vi "ensureLineFeedAfterString.vi"(8 "error in (no error)":errorcluster, 10 "Element":string, 11 "WriteElement in":refnum<class "XMLGenerator.lvclass">) -> (0 "error out":errorcluster, 2 "ElementWithNewLine":string, 3 "WriteElement out":refnum<class "XMLGenerator.lvclass">)   [LabVIEW 2016, in "XML.lvlib" / "XMLGenerator.lvclass"]
doc: "This method seraches the Element in and returns the element back with a line feed."
uses:
  <userlib>/Common/XML/XMLGenerator/XMLGenerator.lvclass
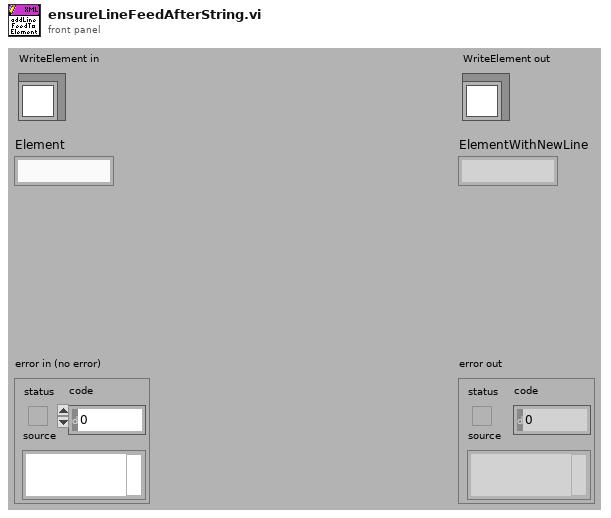
[diagram p1: front panel]
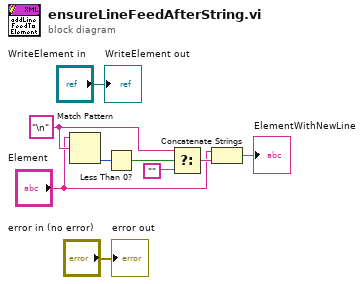
[diagram p0: block diagram]
diagram:
  w3 = "\n" ("regular expression")
  n1 = Match Pattern(string="Element", regular expression=w3) -> (offset past match=w7:i32)  [unwired: 1 in, 3 out]
  n2 = Less Than 0?(x=w7) -> (x < 0?=w6:bool)
  n3 = Select(t=w3, s=w6, f="") -> (s? t:f=w5:string)
  n4 = Concatenate Strings("Element", w5) -> (→"ElementWithNewLine":string)
  "error out" <- "error in (no error)"
  "WriteElement out" <- "WriteElement in"
